vi "Main.vi"() -> ()   [LabVIEW 2017, in "Retrieved Data.lvclass"]
uses:
  Retrieved Data.lvclass
  <vilib>/Utility/miscctls.llb/LVRowAndColumnTypeDef.ctl
  <vilib>/Analysis/NI_AALPro.lvlib
panel:
  in  "Retrieved Data.lvclass":refnum<class "Retrieved Data.lvclass">
  in  "Reset":bool caption="Open"
  in  "Copy to Clipboard":bool caption="Blank"
  in  "Comparison":bool caption="Stop"
  in  "Print":bool
  in  "Info":bool
  in  "Folders to Exclude":string[](array[string]) caption="Folders to exclude"
  in  "Load":bool
  in  "Save":bool caption="Stop"
  in  "Stop":bool
  in  "Pattern":string="??????_B6_SC_#??.txt"
  in  "Folder Path":path=path "C:/Users/KimYG/Desktop" caption="Data File folder 경로"
  in  "Multicol listbox":i32(listbox)
  out "Query result":string[][](table)
  in  "Number of bin":dbl=500.0
  in  "Significant level":enum16{"0.05", "0.01"}(ring)
  in  "Data-set II":u16(ring) items=["??????_B6_VC_#??.txt", "??????_B6_SC_#??.txt"]
  in  "Data-set I":u16(ring) items=["??????_B6_VC_#??.txt", "??????_B6_SC_#??.txt"]
  out "IEI":T1(graph) caption="히스토그램 그래프"
  out "Amplitude":T1(graph) caption="히스토그램 그래프"
  out "P-value":dbl
  out "P-value":dbl
  out "Mean frequency":cluster{dbl[], dbl[]}[](graph)
  out "Mean amplitude":cluster{dbl[], dbl[]}[](graph)
  out "CP_IEI":cluster{"X Values":dbl[], dbl[]}[](graph) caption="히스토그램 그래프"
  out "CP_Amplitude":cluster{"X Values":dbl[], dbl[]}[](graph) caption="히스토그램 그래프"
  # "Minhee Retriever"
  # "Comparison analysis parameter"
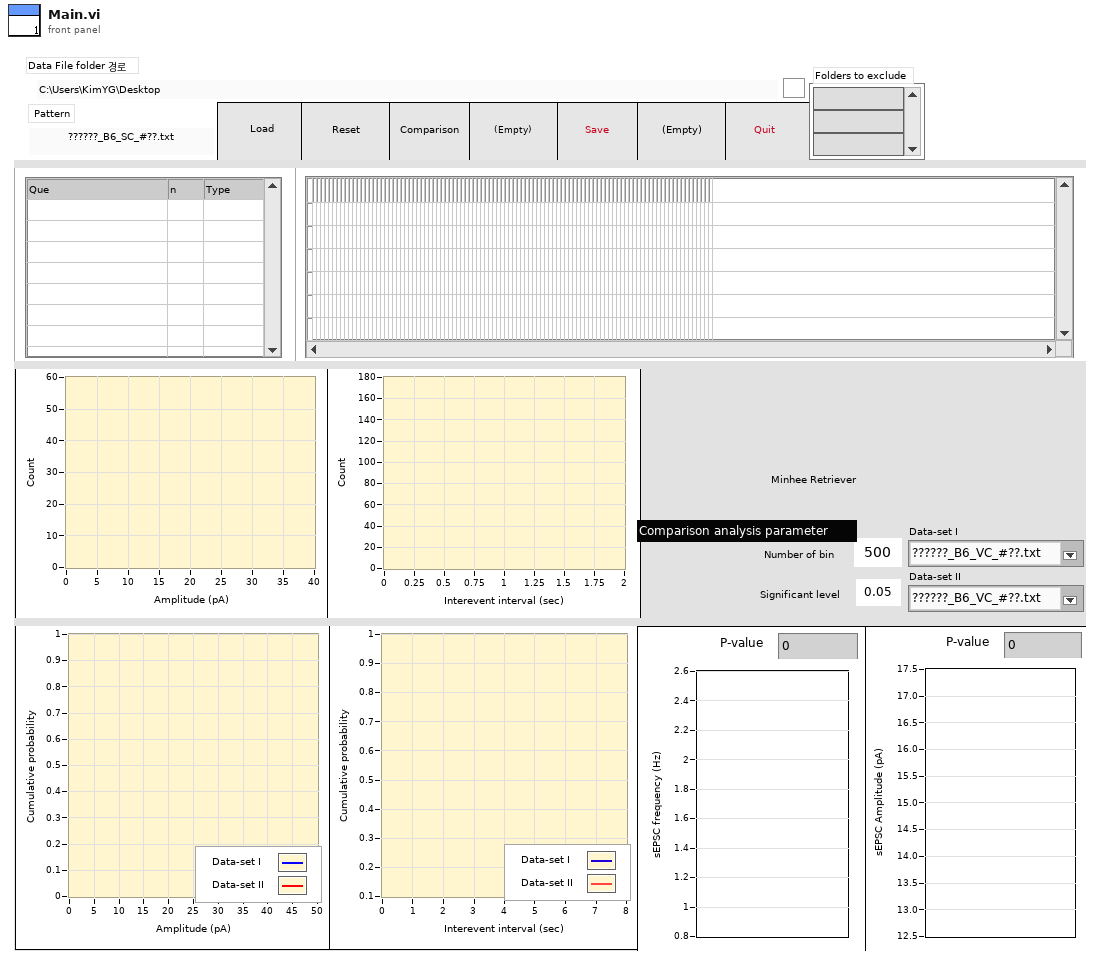
[diagram p1: front panel]
types:
  T1 = cluster{"X Values":dbl[], "Histogram: h(x)":i32[]}
  T2 = typedef "LVRowAndColumnTypeDef.ctl" = cluster{"Row":i32, "Column":i32}
  T3 = cluster{"Folder Path":path, "Pattern":string, "Folders to Exclude":string[]}
  T4 = cluster{"Data-set I":u16, "Data-set II":u16, "Significant level":enum16{"0.05", "0.01"}, "Number of bin":dbl}
  T5 = typedef "Comparison OUT.ctl" = cluster{"CP_Amplitude":cluster{"X Values":dbl[], dbl[]}[], "CP_IEI":cluster{"X Values":dbl[], dbl[]}[], "Mean Amplitude":cluster{dbl[], dbl[]}[], "Mean frequency":cluster{dbl[], dbl[]}[], "t-statistics":cluster{"t-Value":dbl, "DF":i32, "P-value":dbl}[]}
  T6 = cluster{"t-Value":dbl, "DF":i32, "P-value":dbl}[]
  T7 = cluster{"Que":string, "File name":string[], "Summary":string[][], "Input + Mean,SD,SEM":dbl[][], "Amplitude (pA)":dbl[], "IEI (sec)":dbl[], "Colnames":string[], "Rownames":string[]}
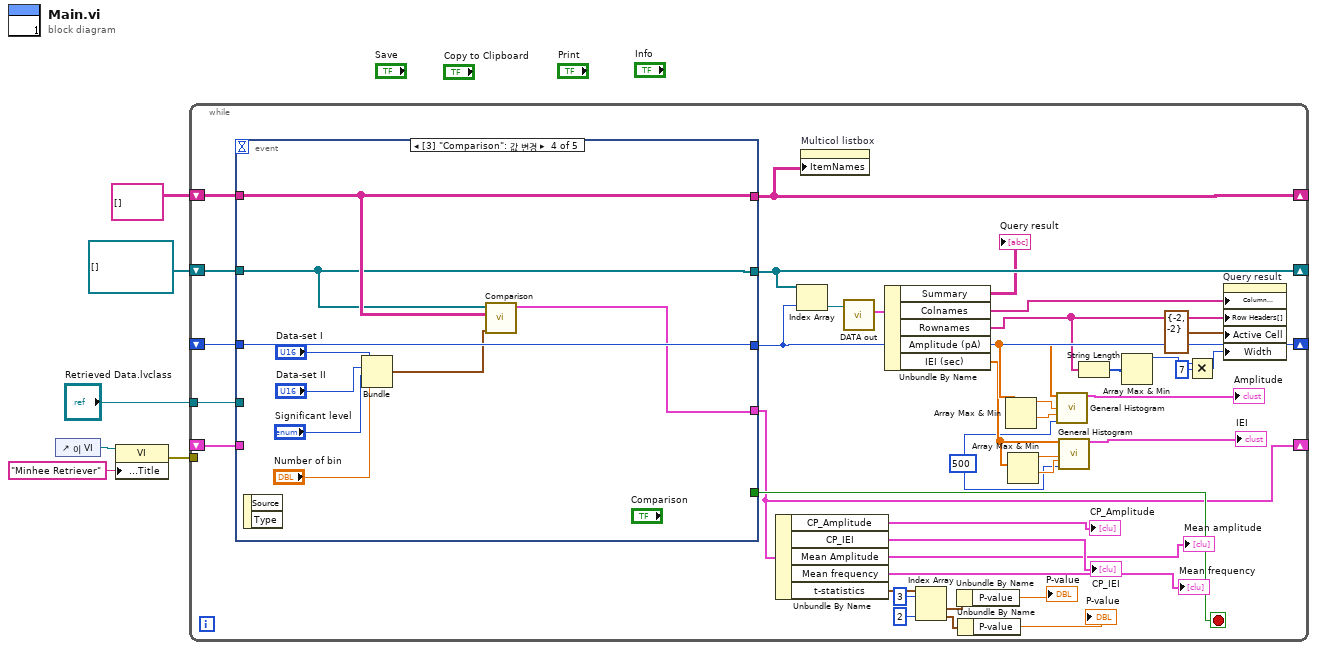
[diagram p0: block diagram]
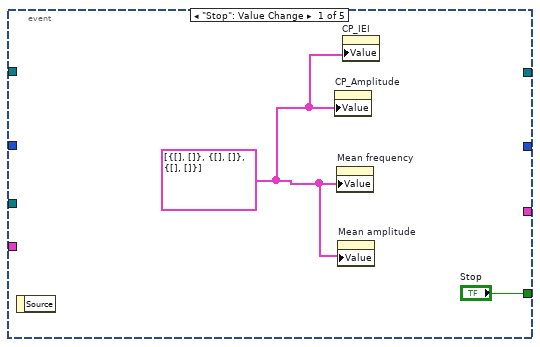
[diagram p2: hidden frame]
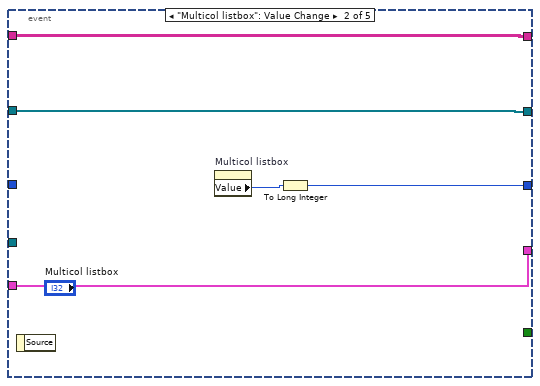
[diagram p3: hidden frame]
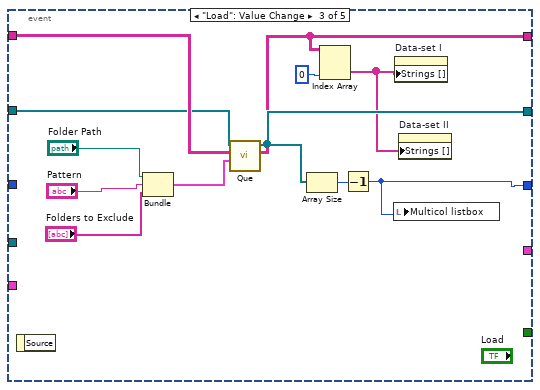
[diagram p4: hidden frame]
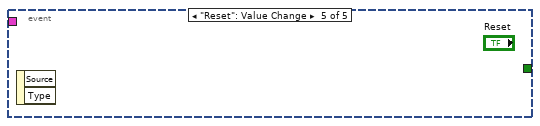
[diagram p5: hidden frame]
diagram:
  n1 = control-ref of="이 VI"() -> (w3:refnum<vi>)
  n2 = property class="VI"(reference=w3, "Front Panel.Title"="Minhee Retriever" ("프런트패널 윈도우:제목")) -> (error out=w1:errorcluster)  [unwired: 1 in, 1 out]
  n3 = while {
    shift-right: [w44] -> _
    shift-left: string[][] [] -> [w45]
    shift-right: [w41] -> _
    shift-left: refnum<class "Retrieved Data.lvclass">[] [] -> [w43]
    shift-right: [w40] -> _
    shift-left: _ -> [w42]
    tunnel: "Retrieved Data.lvclass" -> [w38]
    tunnel: w1 -> [_]
    shift-right: [w7] -> _
    shift-left: _ -> [w25]
    stop <- w46 stop-if-true
    w26 = 500 ("# bins")
    n4 = event shown="[3] \"Comparison\": 값 변경" {
      selector: _ -> [_ _ _ _ _]
      dyn-events: _ -> [_ _ _ _ _]
      timeout: _ -> [_ _ _ _ _]
      tunnel: ["Stop" _ _ _ _] -> w46
      tunnel: w45 -> [_ w53 w59 w73 _]
      tunnel: [_ w53 w55 w73 _] -> w44
      tunnel: w43 -> [_ w50 w58 w72 _]
      tunnel: [_ w50 w57 w72 _] -> w41
      tunnel: [_ w51 w60 w74 _] -> w40
      tunnel: w42 -> [_ _ _ w74 _]
      tunnel: w38 -> [_ _ _ _ _]
      tunnel: [_ w49 _ w66 _] -> w7
      tunnel: w25 -> [_ w49 _ _ _]
      event "Stop": Value Change {
        w47 = cluster{dbl[], dbl[]}[] [{[], []}, {[], []}, {[], []}] ("Mean frequency")
        n5 = event-data() -> ()  [unwired: 1 in, 1 out]
        n6 = property on="CP_Amplitude" class="XYGraph (엄격한)"("Value"=w47) -> ()  [unwired: 2 in, 2 out]
        n7 = property on="Mean frequency" class="XYGraph (엄격한)"("Value"=w47) -> ()  [unwired: 2 in, 2 out]
        n8 = property on="Mean amplitude" class="XYGraph (엄격한)"("Value"=w47) -> ()  [unwired: 2 in, 2 out]
        n9 = property on="CP_IEI" class="XYGraph (엄격한)"("Value"=w47) -> ()  [unwired: 2 in, 2 out]
      }
      event "Multicol listbox": Value Change {
        n10 = event-data() -> ()  [unwired: 1 in, 1 out]
        n11 = property on="Multicol listbox" class="MCListbox (엄격한)"() -> ("Value"=w52:i32)  [unwired: 2 in, 2 out]
        n12 = To Long Integer(number=w52) -> (32bit integer=w51:i32)
      }
      event "Load": Value Change {
        n13 = event-data() -> ()  [unwired: 1 in, 1 out]
        n14 = Bundle("Folder Path"="Folder Path", "Pattern"="Pattern", "Folders to Exclude"="Folders to Exclude") -> (w62:T3)  [unwired: 1 in]
        n15 = call "Que.vi"("Que info"=w62, "Muticol listbox in"=w59, "Data stack IN"=w58) -> ("Muticol listbox out"=w55:string[][], "Data stack OUT"=w57:refnum<class "Retrieved Data.lvclass">[])  [unwired: 2 in, 1 out]
        n16 = Array Size(array=w57) -> (size(s)=w61:i32)
        n17 = Index Array(array=w55, index (col)=0 ("비활성화된 인덱스 (열)")) -> (element=w54:string[])  [unwired: 1 in]
        n18 = Decrement(x=w61) -> (x-1=w60:i32)
        n19 = local write "Multicol listbox"(w60) -> ()
        n20 = property on="Data-set I" class="Ring (엄격한)"("Strings []"=w54) -> ()  [unwired: 2 in, 2 out]
        n21 = property on="Data-set II" class="Ring (엄격한)"("Strings []"=w54) -> ()  [unwired: 2 in, 2 out]
      }
      event "Comparison": Value Change {
        n22 = event-data() -> ()  [unwired: 1 in, 2 out]
        n23 = Bundle("Data-set I"="Data-set I", "Data-set II"="Data-set II", "Significant level"="Significant level", "Number of bin"="Number of bin") -> (w67:T4)  [unwired: 1 in]
        n24 = call "Comparison.vi"("Comparison parameter"=w67, "Muticol listbox IN"=w73, "Data Stack IN"=w72) -> ("Comparison out"=w66:T5)  [unwired: 4 in]
      }
      event "Reset": Value Change {
        n25 = event-data() -> ()  [unwired: 1 in, 2 out]
      }
    }
    n26 = Unbundle By Name(w7) -> ("CP_Amplitude"=→"CP_Amplitude":cluster{"X Values":dbl[], dbl[]}[], "CP_IEI"=→"CP_IEI":cluster{"X Values":dbl[], dbl[]}[], "Mean Amplitude"=→"Mean amplitude":cluster{dbl[], dbl[]}[], "Mean frequency"=→"Mean frequency":cluster{dbl[], dbl[]}[], "t-statistics"=w20:T6)
    n27 = Index Array(array=w41, index=w40) -> (element=w39:refnum<class "Retrieved Data.lvclass">)
    n28 = property on="Multicol listbox" class="MCListbox (엄격한)"("ItemNames"=w44) -> ()  [unwired: 2 in, 2 out]
    n29 = call "DATA out.vi"("Class in"=w39) -> ("Data"=w37:T7)  [unwired: 5 in, 1 out]
    n30 = Unbundle By Name(w37) -> ("Summary"=→"Query result":string[][], "Colnames"=w35:string[], "Rownames"=w13:string[], "Amplitude (pA)"=w32:dbl[], "IEI (sec)"=w29:dbl[])
    n31 = Index Array(array=w20, index #1=3 ("인덱스"), index #2=2 ("인덱스")) -> (element #1=w19:cluster{"t-Value":dbl, "DF":i32, "P-value":dbl}, element #2=w18:cluster{"t-Value":dbl, "DF":i32, "P-value":dbl})
    n32 = Unbundle By Name(w19) -> ("P-value"=→"P-value":dbl)
    n33 = Unbundle By Name(w18) -> ("P-value"=→"P-value":dbl)
    n34 = Array Max & Min(array=w32) -> (max value=w30:dbl, min value=w31:dbl)  [unwired: 2 out]
    n35 = Array Max & Min(array=w29) -> (max value=w28:dbl, min value=w27:dbl)  [unwired: 2 out]
    n36 = call <vilib>:"General Histogram.vi"("X"=w32, "max"=w30, "min"=w31, "# bins"=w26) -> ("Histogram Graph"=→"Amplitude":T1)  [unwired: 7 in, 4 out]
    n37 = call <vilib>:"General Histogram.vi"("X"=w29, "max"=w28, "min"=w27, "# bins"=w26) -> ("Histogram Graph"=→"IEI":T1)  [unwired: 7 in, 4 out]
    n38 = String Length(string=w13) -> (length=w12:i32[])
    n39 = Array Max & Min(array=w12) -> (max value=w11:i32)  [unwired: 3 out]
    n40 = Multiply(x=w11, y=7) -> (x*y=w9:i32)
    n41 = property on="Query result" class="Tbl (엄격한)"("Column Headers[]"=w35, "Row Headers[]"=w13, "Active Cell"=T2 {"Row"=-2, "Column"=-2} ("활성 셀:활성 셀"), "Width"=w9) -> ()  [unwired: 2 in, 2 out]
  }
